vi "GenerateCode.vi"(1 "Terms":T1[](array[typedef]), 3 "Diagram":refnum<vi>, 5 "XRef":refnum<vi>, 6 "State In":T4={"Output Type"=variant(dbl 0.0), "Typedef Name"="", "Input Type"=variant, "Constant Types"=[], "Error"={"status"=FALSE, "code"=0, "source"=""}, "Typedef Path"=path "", "Names"=[], "Event Cluster Name"=""}) -> (0 "Generated Code?":bool, 2 "State Out":T4={"Output Type"=variant(dbl 0.0), "Typedef Name"="", "Input Type"=variant, "Constant Types"=[], "Error"={"status"=FALSE, "code"=0, "source"=""}, "Typedef Path"=path "", "Names"=[], "Event Cluster Name"=""}, 4 "Reply":string[](array[string]))   [LabVIEW 2015, in "Create-Signals.xnode"]
doc: "This ability VI is called when it is time to define the execution behavior of your XNode via LabVIEW's scripting API. This VI is only called when you have previously informed LabVIEW that you need to script through a GenerateCode reply. Diagram is a reference to a diagram of a temporary VI. This diagram contains exactly one front panel terminal for each terminal of your XNode. Terms is an array of pairs of Term IDs and terminal references. LabVIEW will copy code scripted into this diagram into your XNode and connect everything to the correct terminals. The front panel terminals that are on this diagram are special in that they can only be on the top level diagram.\n \n Generate Code? is used to tell LabVIEW whether or not you want to copy the scripted diagram over. If there is an error and you wish not to commit the changes, then the old XNode behavior will be left unchanged. If you set Generate Code? to false, then this VI will be called again next time type propagation is run. Otherwise, it will not be called until you indicate that it should be through the reply on another ability VI.\n \n Because the diagram you are scripting into is separate from the VI containing the XNode instance, type propagation and the data manager will run on the temporary VI after each scripting call.\n \n You should not use the Copy scripting method to move code into the temporary VI. This will adversely affect the user's clipboard. You should use the Move scripting method instead.\n\nDefault behavior: None.\n\nThis ability does not provide UI and OS messages are not handled.\n\nSee also: ModifyCode"
uses:
  Create-Signals.xnode
  State.ctl
  <vilib>/XNodeSupport/XNodeTermIDPair.ctl
  <vilib>/XNodeSupport/XNodeTermRef.ctl
  <vilib>/XNodeSupport/XNodeString.ctl
  <vilib>/LV-Scripting/LV-Scripting.lvlib
  <vilib>/Utility/Data Type/NI_Data Type.lvlib
  <vilib>/XNodeSupport/NI_XNodeSupport.lvlib
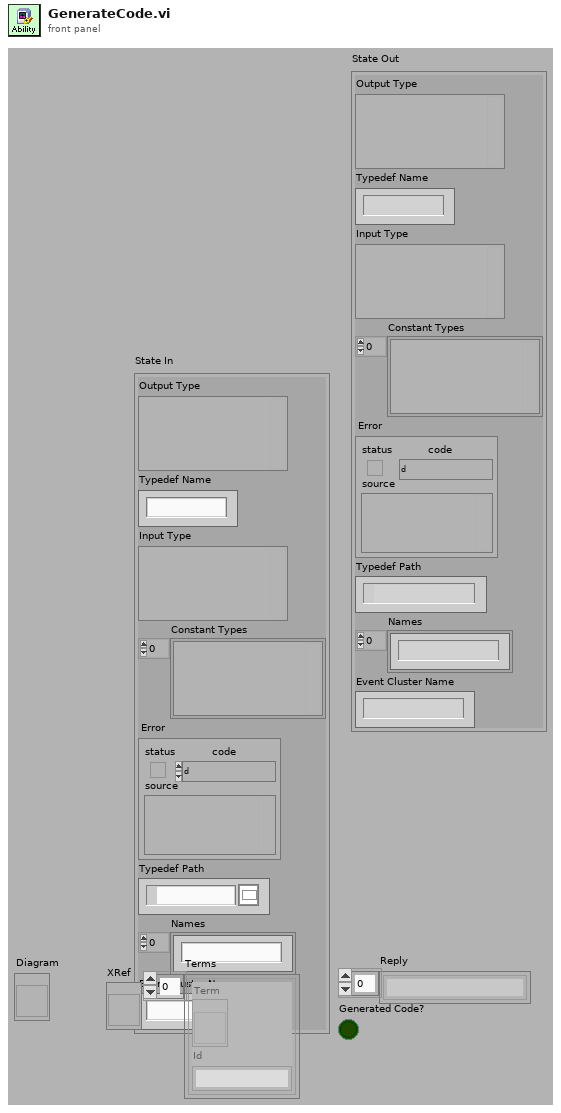
[diagram p1: front panel]
types:
  T1 = typedef "NI_XNodeSupport.lvlib/XNodeTermIDPair.ctl" = cluster{"Term":T2, "Id":T3}
  T2 = typedef "NI_XNodeSupport.lvlib/XNodeTermRef.ctl" = refnum<vi>
  T3 = typedef "NI_XNodeSupport.lvlib/XNodeString.ctl" = string
  T4 = typedef "Create-Signals.xnode/State.ctl" = cluster{"Output Type":variant, "Typedef Name":string, "Input Type":variant, "Constant Types":variant[], "Error":errorcluster, "Typedef Path":path, "Names":string[], "Event Cluster Name":string}
  T5 = typedef "NI_Data Type.lvlib/Type Definition Info.ctl" = cluster{"Name":string, "Timestamp":u32}
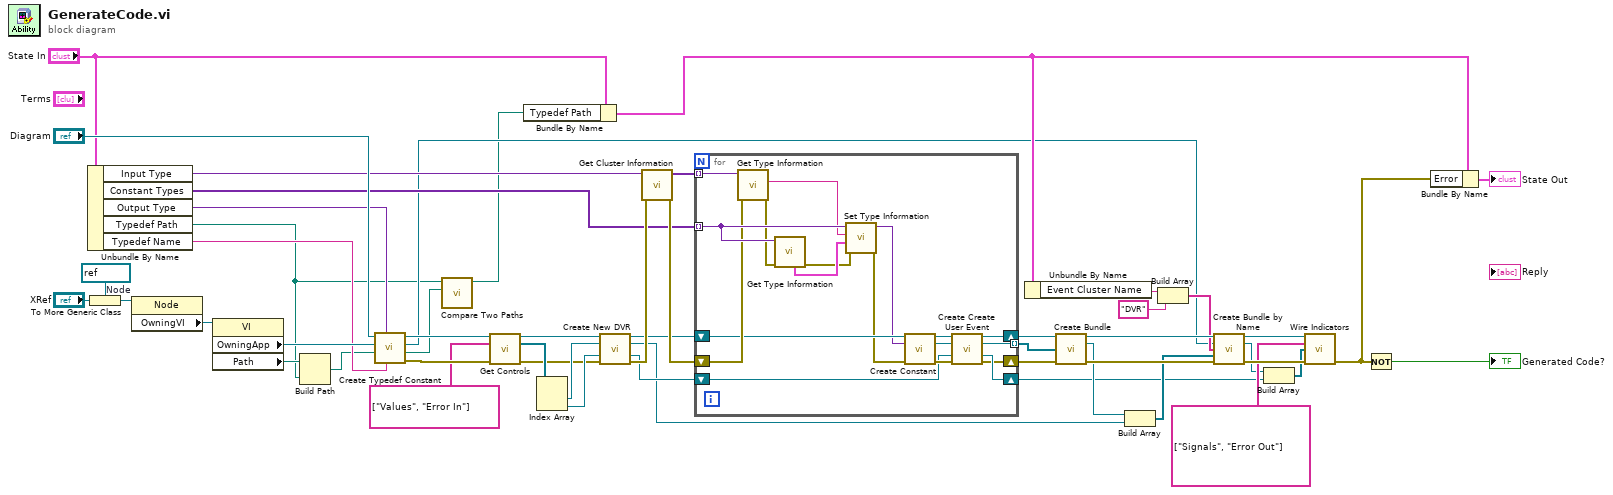
[diagram p0: block diagram]
diagram:
  w51 = refnum<vi> refnum  # Node
  n1 = Unbundle By Name("State In") -> ("Input Type"=w32:variant, "Constant Types"=w31:variant[], "Output Type"=w45:variant, "Typedef Path"=w3:path, "Typedef Name"=w44:string)
  n2 = To More Generic Class(target class=w51, reference="XRef") -> (generic class reference=w50:refnum<vi>)
  n3 = property class="Node"(reference=w50) -> ("OwningVI"=w49:refnum<vi>)  [unwired: 1 in, 2 out]
  n4 = property class="VI"(reference=w49) -> ("OwningApp"=w47:refnum<vi>, "Path"=w5:path)  [unwired: 1 in, 2 out]
  n5 = Build Path(base path=w5, name or relative path=w3) -> (appended path=w4:path)
  n6 = call <vilib>:"Create Typedef Constant.vi"("Typedef Name"=w44, "Type"=w45, "Typedef Path"=w4, "Application"=w47, "Diagram in"="Diagram") -> ("error out"=w42:errorcluster, "New Typedef Path"=w2:path, "Constant"=w6:refnum<vi>, "Diagram out"=w43:refnum<vi>)  [unwired: 3 in]
  n7 = call <vilib>:"Compare Two Paths.vi"("Path 2"=w2, "Path 1"=w3) -> ("Relative Path from 1 to 2"=w1:path)  [unwired: 6 in, 3 out]
  n8 = call <vilib>:"Get Controls.vi"("Diagram in"=w43, "Control Names"=string[] ["Values", "Error In"], "error in (no error)"=w42) -> ("Diagram out"=w39:refnum<vi>, "Control Terminals"=w40:refnum<vi>[], "error out"=w36:errorcluster)  [unwired: 10 in]
  n9 = Bundle By Name(cluster="State In", "Typedef Path"=w1) -> (w13:T4)
  n10 = Index Array(array=w40) -> (element #1=w38:refnum<vi>, element #2=w37:refnum<vi>)  [unwired: 2 in]
  n11 = call <vilib>:"Create New DVR.vi"("Diagram in"=w39, "data value"=w38, "error in"=w37, "error in (no error)"=w36) -> ("Diagram out"=w30:refnum<vi>, "data value reference"=w19:refnum<vi>, 10:"error out"=w29:refnum<vi>, 15:"error out"=w33:errorcluster)  [unwired: 8 in]
  n12 = call <vilib>:"Get Cluster Information.vi"("error in (no error)"=w33, "Variant"=w32) -> ("error out"=w34:errorcluster, "Cluster Elements"=w35:variant[])  [unwired: 8 in]
  n13 = for {
    shift-right: [w52] -> w26
    shift-left: w34 -> [w65]
    shift-right: [w53] -> w27
    shift-left: w30 -> [w62]
    shift-right: [w55] -> w8
    shift-left: w29 -> [w57]
    tunnel: [w54] -> w28 mode=indexing
    tunnel: w31 -> [w69] mode=indexing
    tunnel: w35 -> [w66] mode=indexing
    n14 = call <vilib>:"Get Type Information.vi"("error in (no error)"=w65, "Variant"=w66) -> ("error out"=w64:errorcluster, "Name"=w63:string)  [unwired: 5 in, 3 out]
    n15 = call <vilib>:"Get Type Information.vi"("error in (no error)"=w64, "Variant"=w69) -> ("error out"=w67:errorcluster, "Type Definition Info"=w68:T5)  [unwired: 5 in, 3 out]
    n16 = call <vilib>:"Set Type Information.vi"("error in (no error)"=w67, "Type Definition Info"=w68, "Name"=w63, "Variant in"=w69) -> ("error out"=w61:errorcluster, "Variant out"=w60:variant)  [unwired: 6 in]
    n17 = call <vilib>:"Create Constant.vi"("Diagram in"=w62, "Type"=w60, "error in (no error)"=w61) -> ("Diagram out"=w59:refnum<vi>, "Terminal"=w56:refnum<vi>, "error out"=w58:errorcluster)  [unwired: 10 in]
    n18 = call <vilib>:"Create Create User Event.vi"("Diagram in"=w59, "user event datatype"=w56, "error in"=w57, "error in (no error)"=w58) -> ("Diagram out"=w53:refnum<vi>, "user event"=w54:refnum<vi>, 10:"error out"=w55:refnum<vi>, 15:"error out"=w52:errorcluster)  [unwired: 8 in]
  }
  n19 = Unbundle By Name(w13) -> ("Event Cluster Name"=w23:string)
  n20 = call <vilib>:"Create Bundle.vi"("Diagram in"=w27, "Inputs"=w28, "error in (no error)"=w26) -> ("Diagram out"=w25:refnum<vi>, "output cluster"=w20:refnum<vi>, "error out"=w24:errorcluster)  [unwired: 10 in]
  n21 = Build Array(w20, w19) -> (w18:refnum<vi>[])
  n22 = Build Array(w23, "DVR" ("element")) -> (w21:string[])
  n23 = call <vilib>:"Create Bundle by Name.vi"("Diagram in"=w25, "input cluster"=w6, "Element Names"=w21, "Inputs"=w18, "error in (no error)"=w24) -> ("Diagram out"=w10:refnum<vi>, "output cluster"=w9:refnum<vi>, "error out"=w16:errorcluster)  [unwired: 8 in]
  n24 = Build Array(w9, w8) -> (w7:refnum<vi>[])
  n25 = call <vilib>:"Wire Indicators.vi"("Diagram in"=w10, "Indicator Names"=string[] ["Signals", "Error Out"], "Outputs"=w7, "error in (no error)"=w16) -> ("error out"=w12:errorcluster)  [unwired: 10 in, 1 out]
  n26 = Not(x=w12) -> (.not. x?=→"Generated Code?":bool)
  n27 = Bundle By Name(cluster=w13, "Error"=w12) -> (→"State Out":T4)
